vi "Write.vi"(8 "error in (no error)":errorcluster, 10 "Write Buffer":string, 11 "VISA resource name":refnum<visa-resource-name>) -> (0 "error out":errorcluster, 3 "VISA resource name out":refnum<visa-resource-name>)   [LabVIEW 2018, in "LeCroy Wave Series.lvlib"]
doc: "Writes data from write buffer to the device or interface specified by VISA resource name. It is modified for beater device communication over TCP/IP.\n\n<B>Note:</B>\n\nThis is a low-level Write VI that can be used to send commands to the instrument for functionality not supported by the driver."
uses:
  LeCroy Wave Series.lvlib
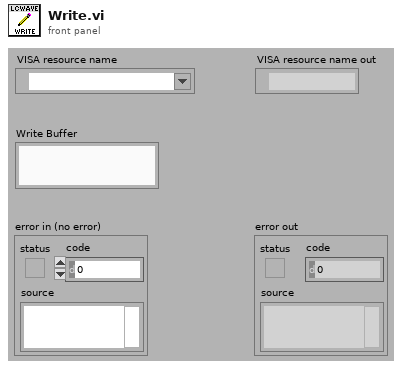
[diagram p1: front panel]
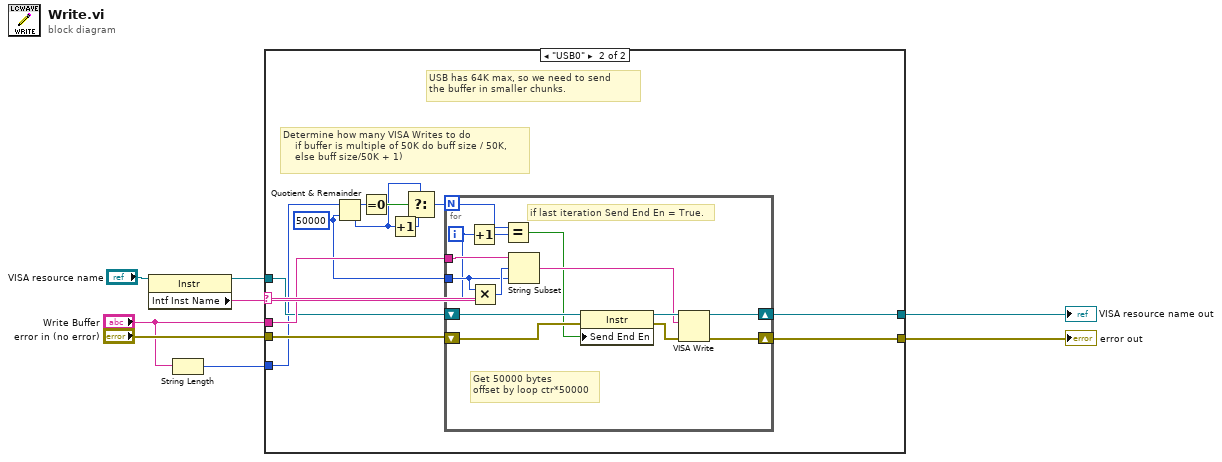
[diagram p0: block diagram]
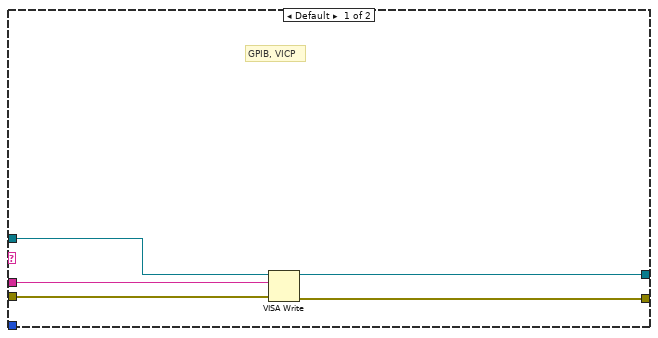
[diagram p2: hidden frame]
diagram:
  n1 = property class="Instr"(reference="VISA resource name") -> (reference out=w4:refnum<visa-resource-name>, "Intf Inst Name"=w3:string)  [unwired: 1 in, 1 out]
  n2 = String Length(string="Write Buffer") -> (length=w1:i32)
  n3 = case shown="\"USB0\"" w3 {
    tunnel: "Write Buffer" -> [w13 w25]
    tunnel: [w12 w24] -> w8
    tunnel: [w11 w23] -> w7
    tunnel: "error in (no error)" -> [w10 w22]
    tunnel: w4 -> [w9 w21]
    tunnel: w1 -> [_ w19]
    frame Default {
      # "GPIB, VICP"
      n4 = VISA Write(VISA resource name=w9, write buffer=w13, error in (no error)=w10) -> (VISA resource name out=w11:refnum<visa-resource-name>, error out=w12:errorcluster)  [unwired: 1 out]
    }
    frame "USB0" {
      w20 = 50000 ("length (rest)")
      # "USB has 64K max, so we need to send\nthe buffer in smaller chunks."
      # "Determine how many VISA Writes to do\n    if buffer is multiple of 50K do buff size / 50K,\n    else buff size/50K + 1)"
      n5 = Quotient & Remainder(x=w19, y=w20) -> (x-y*floor(x/y)=w17:i32, floor(x/y)=w16:i32)
      n6 = Equal To 0?(x=w17) -> (x = 0?=w18:bool)
      n7 = Increment(x=w16) -> (x+1=w15:i32)
      n8 = Select(t=w16, s=w18, f=w15) -> (s? t:f=w14:i32)
      n9 = for {
        N: w14 -> [w30]
        shift-right: [w33] -> w24
        shift-left: w22 -> [w34]
        tunnel: w25 -> [w37]
        tunnel: w20 -> [w35]
        shift-right: [w39] -> w23
        shift-left: w21 -> [w38]
        i -> [w29]
        # "Get 50000 bytes\noffset by loop ctr*50000"
        # "if last iteration Send End En = True."
        n10 = Increment(x=w29) -> (x+1=w28:i32)
        n11 = Multiply(x=w35, y=w29) -> (x*y=w36:i32)
        n12 = Equal?(x=w30, y=w28) -> (x = y?=w26:bool)
        n13 = String Subset(string=w37, offset (0)=w36, length (rest)=w35) -> (substring=w27:string)
        n14 = property class="Instr"(reference=w38, error in=w34, "Send End En"=w26) -> (reference out=w32:refnum<visa-resource-name>, error out=w31:errorcluster)
        n15 = VISA Write(VISA resource name=w32, write buffer=w27, error in (no error)=w31) -> (VISA resource name out=w39:refnum<visa-resource-name>, error out=w33:errorcluster)  [unwired: 1 out]
      }
    }
  }
  "error out" <- w8
  "VISA resource name out" <- w7
